vi "N2.vi"() -> ()   [LabVIEW 2020]
panel:
  in  "Numeric":dbl
  out "Answer":dbl
  in  "degree":i32
  in  "?":bool
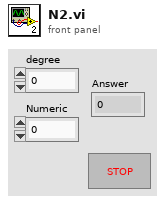
[diagram p1: front panel]
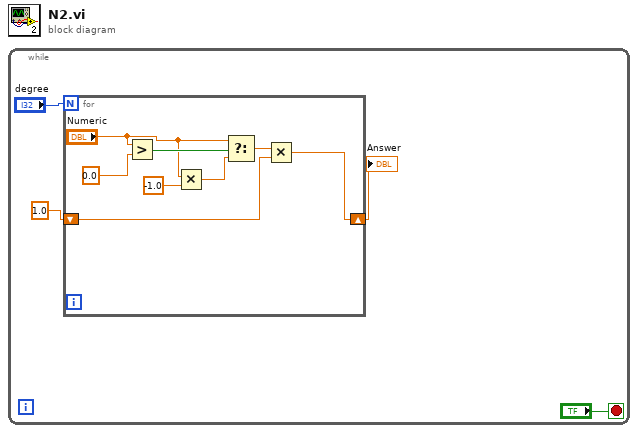
[diagram p0: block diagram]
diagram:
  n1 = while {
    stop <- "?" stop-if-true
    n2 = for {
      N: "degree" -> [_]
      shift-right: [w11] -> w2
      shift-left: 1.0 -> [w12]
      n3 = Greater?(x="Numeric", y=0.0 ("x")) -> (0:w8:bool)
      n4 = Multiply(x="Numeric", y=-1.0) -> (x*y=w6:dbl)
      n5 = Select(t="Numeric", s=w8, f=w6) -> (s? t:f=w10:dbl)
      n6 = Multiply(x=w10, y=w12) -> (x*y=w11:dbl)
    }
    "Answer" <- w2
  }
